vi "UART FGV.vi"(7 "input cluster":T1 {"termination char\n(0xA = '\\n' = LF)" format="%.0x"; "flow control (0:none)" items=["None", "XON/XOFF", "RTS/CTS", "XON/XOFF & RTS/CTS", "DTR/DSR", "XON/XOFF & DTR/DSR"]; "stop bits (10: 1 bit)" items=["1.0"=10, "1.5"=15, "2.0"=20]; "data bits (8)" min=5 max=8 step=1}, 8 "error in (no error)":errorcluster, 9 "error? in":bool, 10 "Read mode":enum16{"Read all", "Get latest value"}(ring)=enum."Get latest value", 11 "VISA Refnum in":refnum<visa-resource-name>) -> (0 "error out":errorcluster, 1 "error? out":bool, 2 "read buffer":string, 3 "timeout (10sec)":u32)   [LabVIEW 2017]
uses:
  <vilib>/myRIO/Instrument Drivers/Onboard IO/UART/typedef/VISA Configuration.ctl
  <vilib>/myRIO/Instrument Drivers/Onboard IO/UART/UART.lvlib
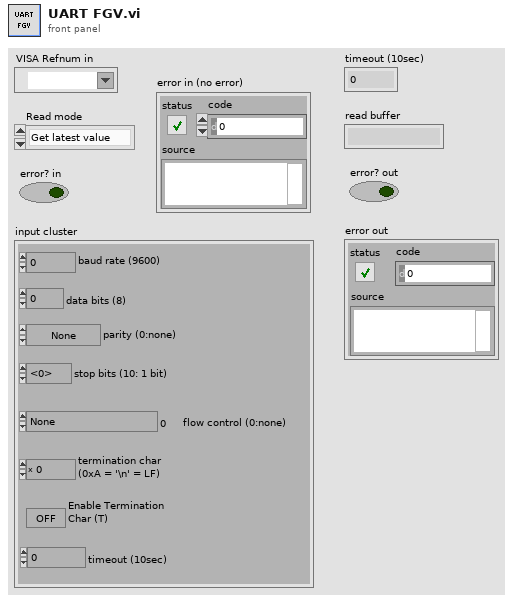
[diagram p1: front panel]
types:
  T1 = typedef "UART.lvlib/VISA Configuration.ctl" = cluster{"baud rate (9600)":u32, "data bits (8)":u16, "parity (0:none)":enum16{"None", "Odd", "Even", "Mark", "Space"}, "stop bits (10: 1 bit)":u16, "flow control (0:none)":u16, "termination char\n(0xA = '\\n' = LF) ":u8, "Enable Termination\nChar (T)":bool, "timeout (10sec)":u32}
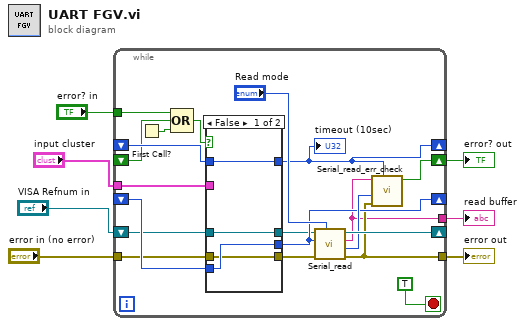
[diagram p0: block diagram]
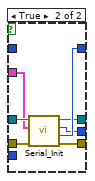
[diagram p2: hidden frame]
diagram:
  n1 = while {
    shift-right: [w26] -> _
    shift-left: "VISA Refnum in" -> [w18]
    shift-right: [w23] -> _
    shift-left: _ -> [w22]
    shift-right: [w21] -> _
    shift-left: _ -> [w20]
    tunnel: "input cluster" -> [w15]
    tunnel: [w14] -> w5
    tunnel: [w13] -> w6
    tunnel: "error in (no error)" -> [w12]
    shift-right: [w16] -> w7
    shift-left: _ -> [w9]
    tunnel: "error? in" -> [w11]
    stop <- TRUE stop-if-true
    n2 = First Call?() -> (First Call?: T/F=w10:bool)
    n3 = Compound Arithmetic op=OR(w11, w9, w10) -> (w8:bool)
    n4 = case shown="False" w8 {
      tunnel: [w28 w38] -> w24
      tunnel: [w30 w37] -> w21
      tunnel: [w31 w36] -> w23
      tunnel: w22 -> [w31 _]
      tunnel: w20 -> [w30 _]
      tunnel: [w29 w35] -> w19
      tunnel: w18 -> [w29 w34]
      tunnel: w15 -> [_ w33]
      tunnel: w12 -> [w28 w32]
      frame False {
      }
      frame True {
        n5 = call "Serial_Init.vi"("error in (no error)"=w32, "input cluster"=w33, "VISA Refnum in"=w34) -> ("error out"=w38:errorcluster, "timeout (10sec)"=w37:u32, "Bytes at Port"=w36:u32, "VISA Refnum out"=w35:refnum<visa-resource-name>)  [unwired: 5 in]
      }
    }
    "timeout (10sec)" <- w21
    n6 = call "Serial_read.vi"("Read mode"="Read mode", "error in (no error)"=w24, "Bytes at Port"=w23, "VISA Refnum in"=w19) -> ("error out"=w14:errorcluster, "dt"=w25:u32, "read buffer"=w13:string, "VISA resource name out"=w26:refnum<visa-resource-name>)  [unwired: 4 in]
    n7 = call "Serial_read_err_check.vi"("timeout"=w21, "error in (no error)"=w14, "dt"=w25, "read buffer"=w13) -> ("error?"=w16:bool)  [unwired: 7 in]
  }
  "error? out" <- w7
  "read buffer" <- w6
  "error out" <- w5
